vi "nirviSubSaturate.vi"(1 "y":i32, 2 "x":i32) -> (0 "x-y":i32)   [LabVIEW 2017]
doc: "Computes the difference between two 32-bit numbers using saturation arithmetic to avoid integer overflow by returning a maximum or minimum value."
uses:
  <vilib>/rvi/Arithmetic/AddSubMult/XNode/nirviSatArithmetic.xnode
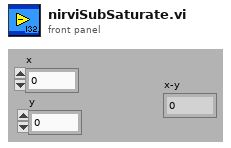
[diagram p1: front panel]
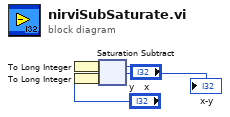
[diagram p0: block diagram]
diagram:
  n1 = To Long Integer(number="x") -> (32bit integer=w1:i32)
  n2 = To Long Integer(number="y") -> (32bit integer=w2:i32)
  n3 = xnode "Saturation Subtract"("x"=w1, "y"=w2) -> ("x-y"=→"x-y":i32)
